vi "loadHTOutcounterOnly.vi"(10 "file path (dialog if empty)":path) -> ()   [LabVIEW 2012]
uses:
  <vilib>/addons/database/Connection.llb/DB Tools Open Connec (Path).vi
  <vilib>/Utility/file.llb/Read From Spreadsheet File (string).vi
  <vilib>/addons/database/Connection.llb/Conn Execute.vi
  <vilib>/addons/database/Recordset.llb/Rec Fetch Integer Data (R).vi
  <vilib>/addons/database/Recordset.llb/Rec Destroy - Connection.vi
  <vilib>/addons/database/NI_Database_API.lvlib
panel:
  out "ToRunSite":string
  out "error out 2":errorcluster
  in  "input cluster":T1
  out "output cluster":T1
  out "SQLDateTime":string
  out "time stamp":timestamp
  out "SQLDateTime 2":string
  out "concatenated string":string
  out "all rows":string[][](array[string])
  out "size(s)":i32[](array[numeric])
  out "output cluster 2":T2
  in  "input cluster 2":T2
  out "before substring 5":string
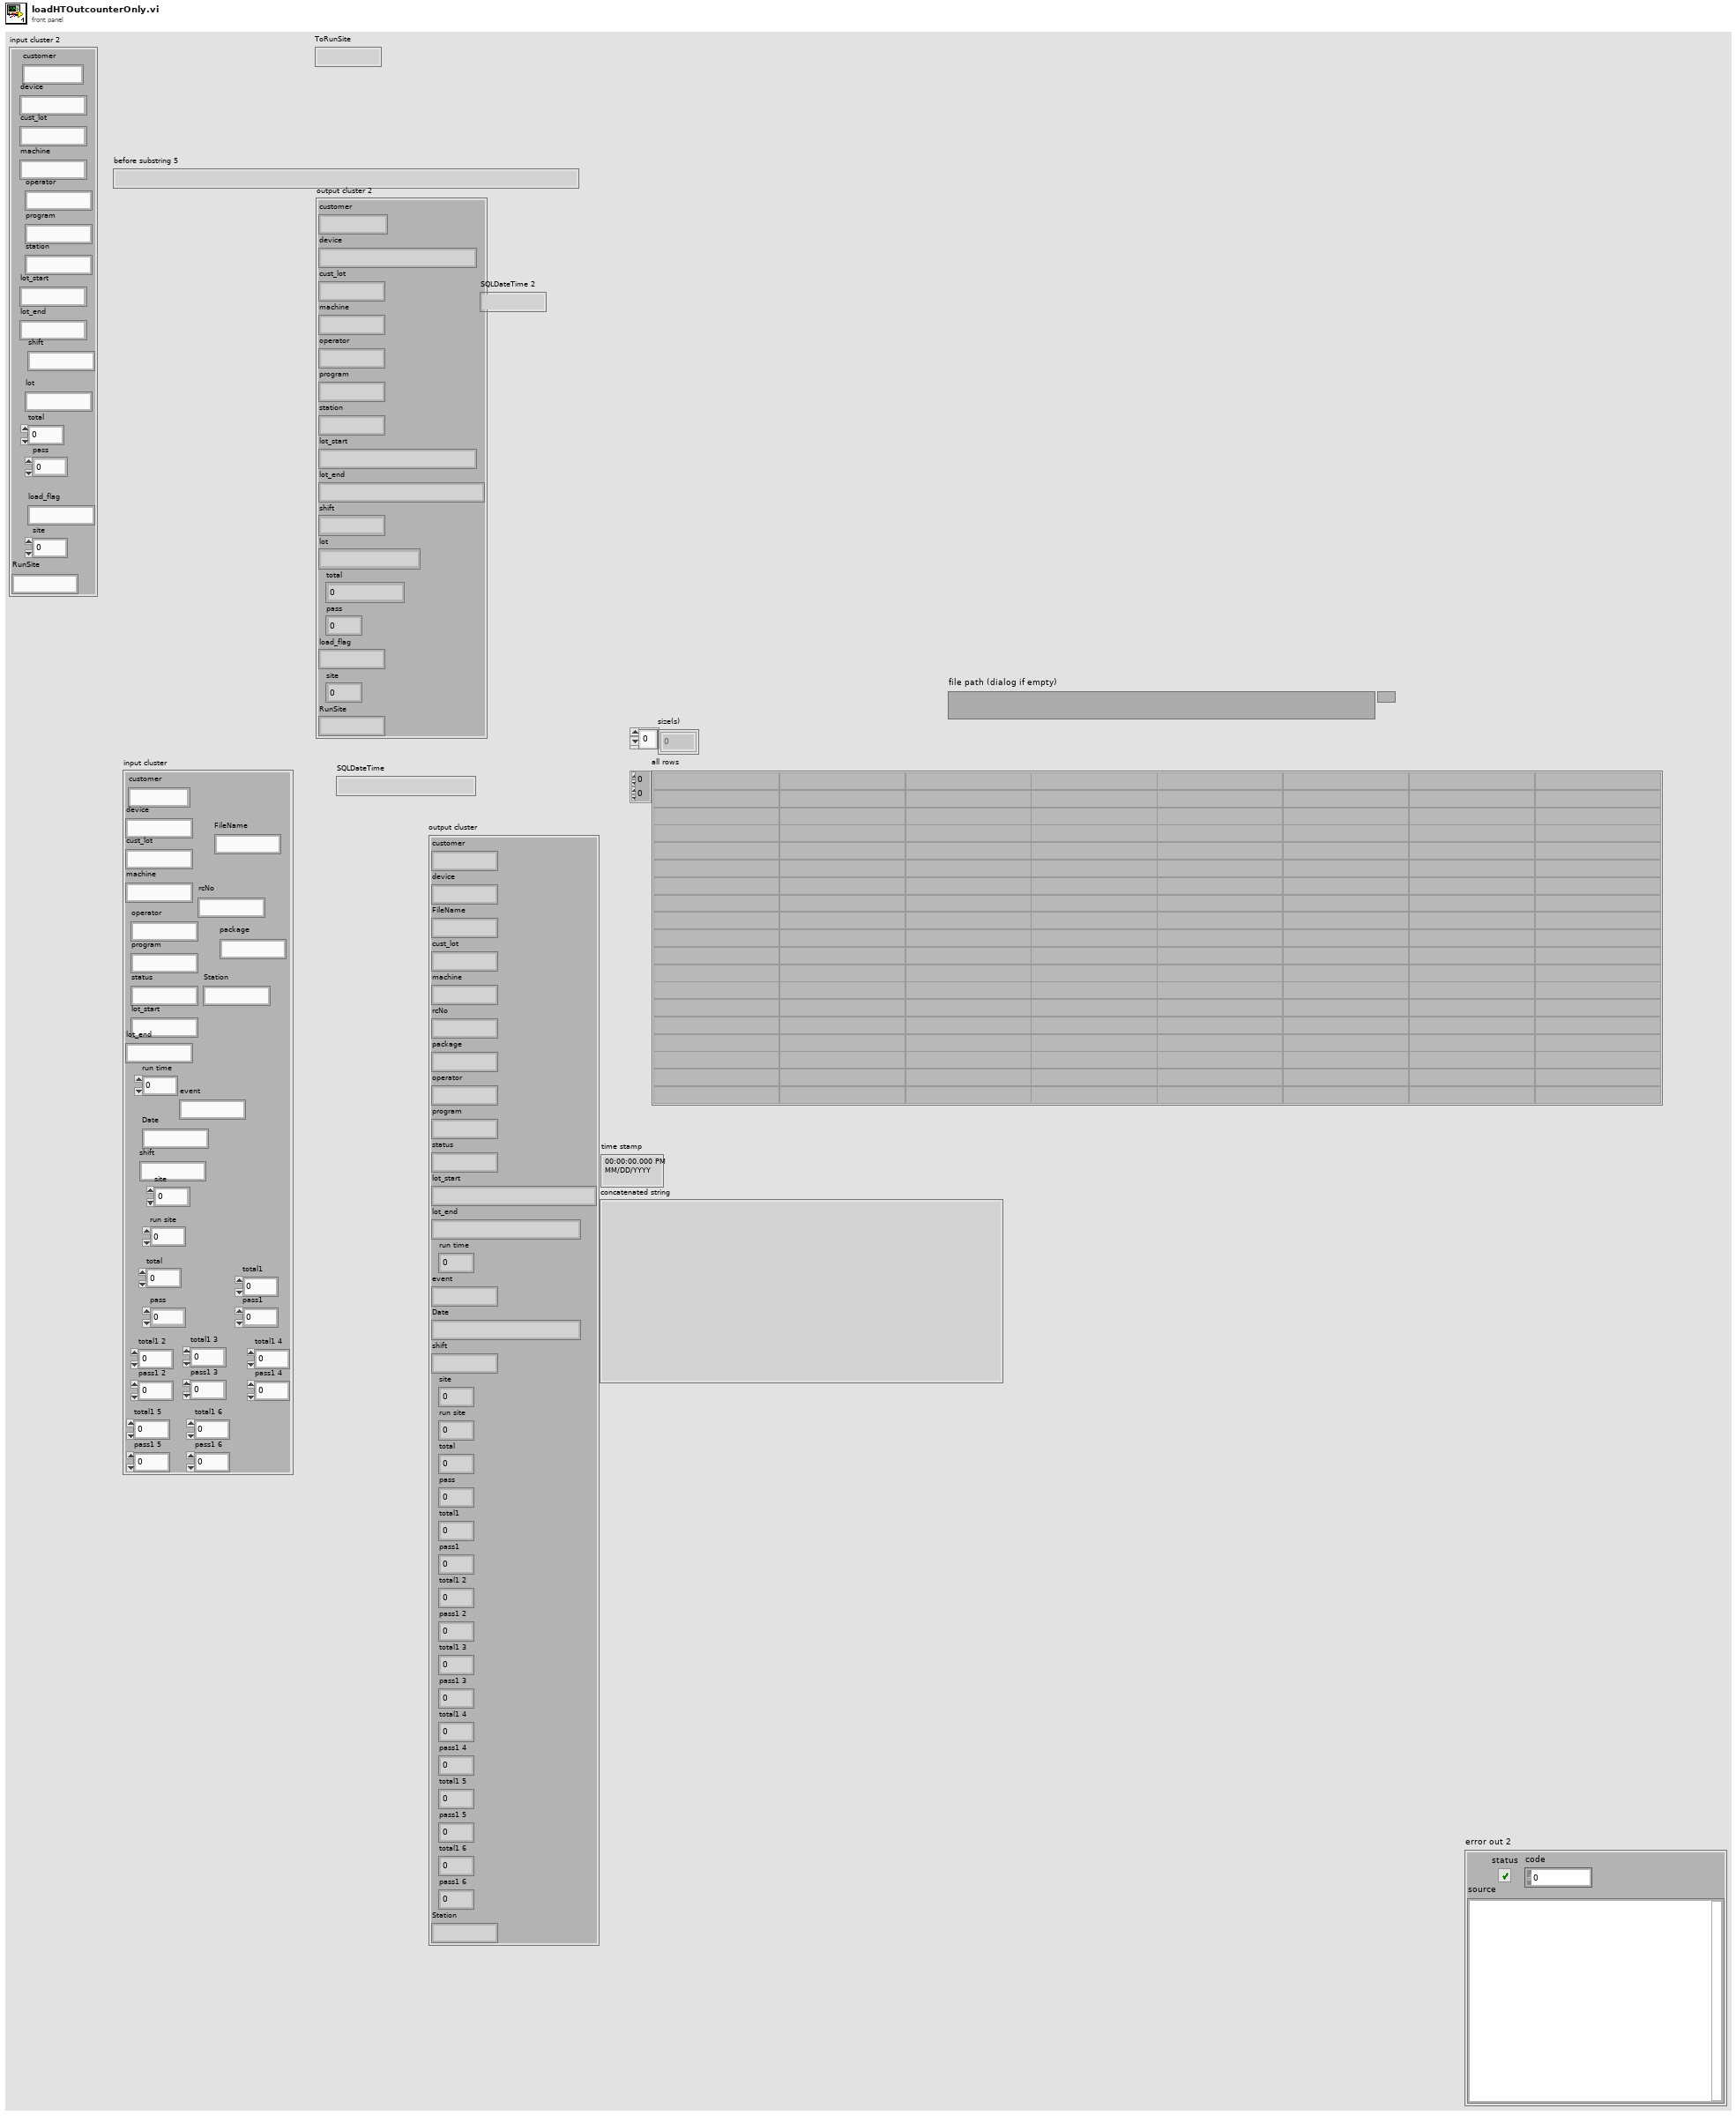
[diagram p1: front panel]
types:
  T1 = cluster{"customer":string, "device":string, "FileName":string, "cust_lot":string, "machine":string, "rcNo":string, "package":string, "operator":string, "program":string, "status":string, "lot_start":string, "lot_end":string, "run time":dbl, "event":string, "Date":string, "shift":string, "site":dbl, "run site ":dbl, "total":dbl, "pass":dbl, "total1":dbl, "pass1":dbl, "total1 2":dbl, "pass1 2":dbl, "total1 3":dbl, "pass1 3":dbl, "total1 4":dbl, "pass1 4":dbl, "total1 5":dbl, "pass1 5":dbl, "total1 6":dbl, "pass1 6":dbl, "Station":string}
  T2 = cluster{"customer":string, "device":string, "cust_lot":string, "machine":string, "operator":string, "program":string, "station":string, "lot_start":string, "lot_end":string, "shift":string, "lot":string, "total":dbl, "pass":dbl, "load_flag":string, "site":dbl, "RunSite":string}
  T3 = typedef "NI_Database_API.lvlib/Conn ObjectReference.ctl" = refnum<k1>
  T4 = typedef "NI_Database_API.lvlib/Rec ObjectReference.ctl" = refnum<k1>
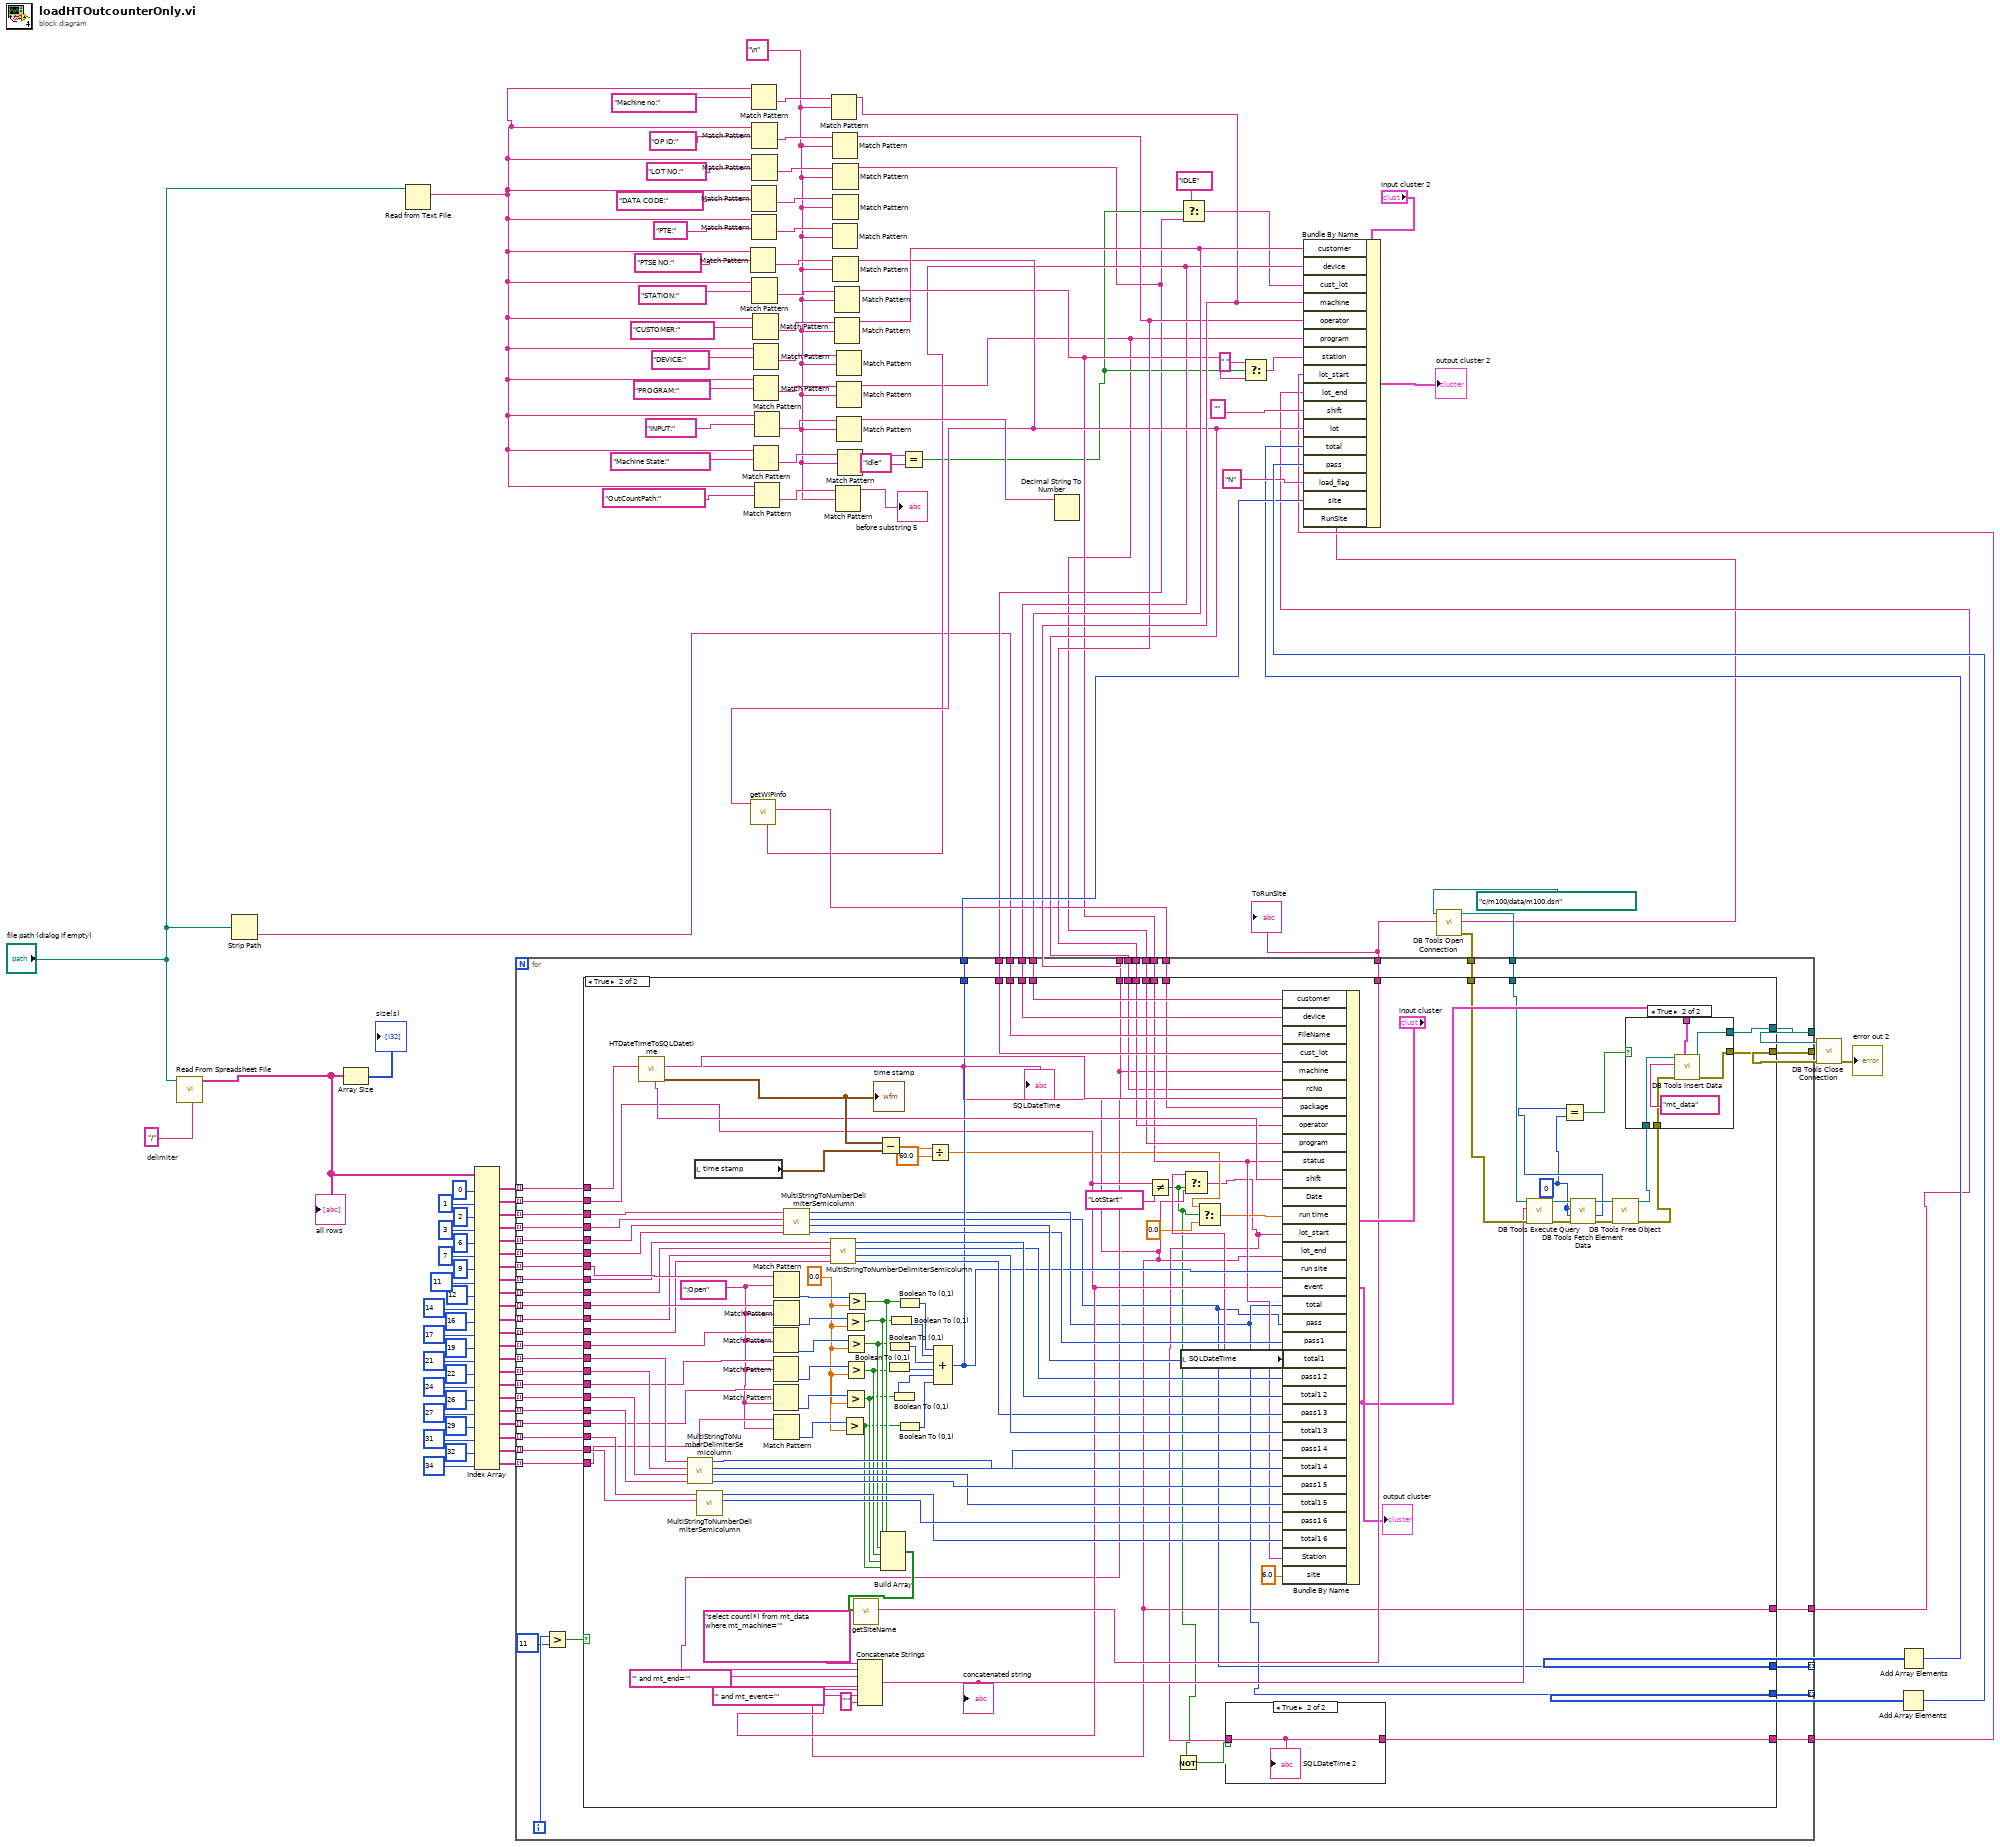
[diagram p0: block diagram]
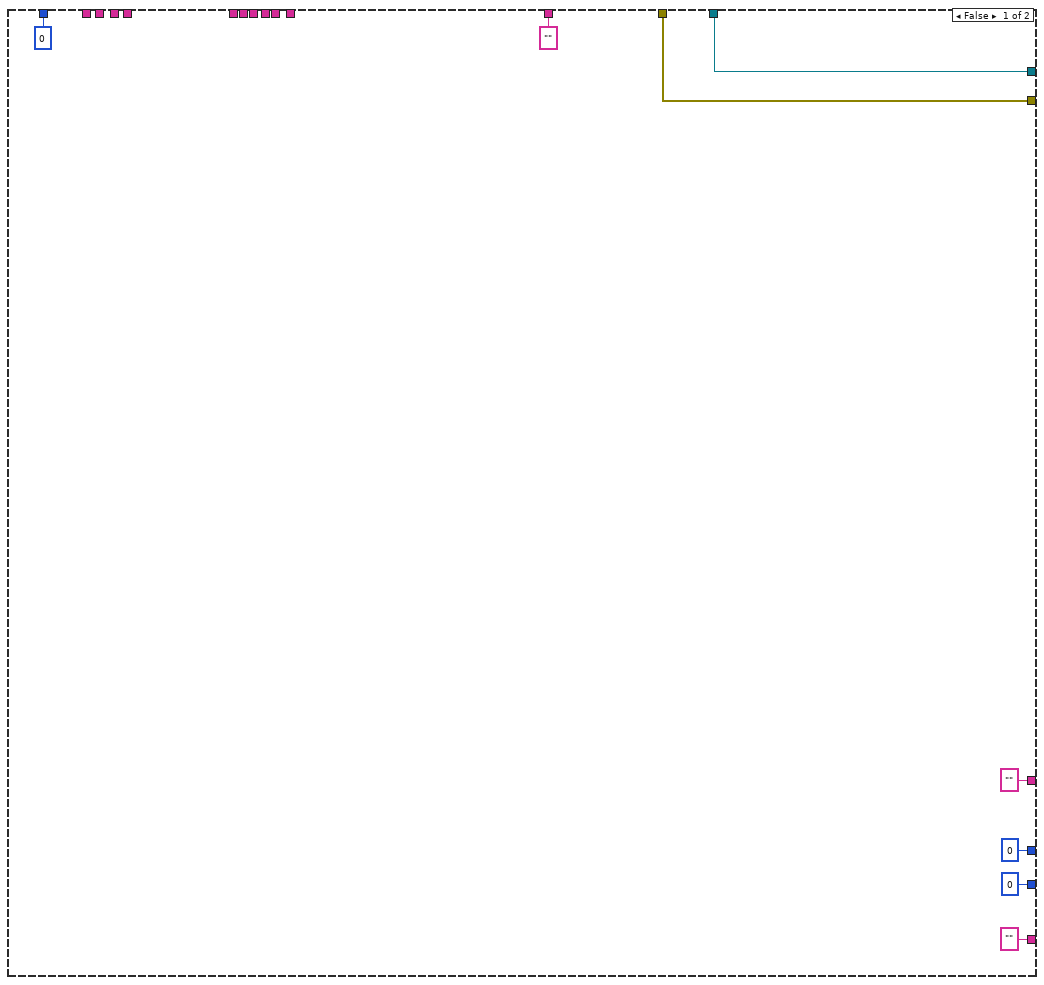
[diagram p2: hidden frame]
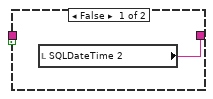
[diagram p4: hidden frame]
diagram:
  w80 = "/"  # delimiter
  w83 = "\n" ("regular expression")
  n1 = call-poly <vilib>:"Read From Spreadsheet File.vi"("delimiter (\\t)"=w80, "file path (dialog if empty)"="file path (dialog if empty)") -> ("all rows"=w78:string[][])  [unwired: 5 in, 4 out]
  "all rows" <- w78
  n2 = Strip Path(path="file path (dialog if empty)") -> (name=w2:string)  [unwired: 1 out]
  n3 = Array Size(array=w78) -> (size(s)=→"size(s)":i32[])
  n4 = Read from Text File(file (use dialog)="file path (dialog if empty)") -> (text=w81:string)  [unwired: 3 in, 3 out]
  n5 = Index Array(array=w78, index (col) #1=0 ("disabled index (col)"), index (col) #2=1 ("index (col)"), index (col) #3=2 ("index (col)"), index (col) #4=3 ("index (col)"), index (col) #5=6 ("index (col)"), index (col) #6=7 ("index (col)"), index (col) #7=9 ("index (col)"), index (col) #8=11 ("index (col)"), index (col) #9=12 ("index (col)"), index (col) #10=14 ("index (col)"), index (col) #11=16 ("index (col)"), index (col) #12=17 ("index (col)"), index (col) #13=19 ("index (col)"), index (col) #14=21 ("index (col)"), index (col) #15=22 ("index (col)"), index (col) #16=24 ("index (col)"), index (col) #17=26 ("index (col)"), index (col) #18=27 ("index (col)"), index (col) #19=29 ("index (col)"), index (col) #20=31 ("index (col)"), index (col) #21=32 ("index (col)"), index (col) #22=34 ("index (col)")) -> (element #1=w76:string[], element #2=w74:string[], element #3=w71:string[], element #4=w70:string[], element #5=w67:string[], element #6=w66:string[], element #7=w64:string[], element #8=w61:string[], element #9=w60:string[], element #10=w58:string[], element #11=w55:string[], element #12=w54:string[], element #13=w52:string[], element #14=w49:string[], element #15=w48:string[], element #16=w46:string[], element #17=w43:string[], element #18=w42:string[], element #19=w40:string[], element #20=w37:string[], element #21=w36:string[], element #22=w34:string[])  [unwired: 22 in]
  n6 = Match Pattern(string=w81, regular expression="PTSE NO:") -> (after substring=w104:string)  [unwired: 1 in, 3 out]
  n7 = Match Pattern(string=w81, regular expression="Machine no:") -> (after substring=w84:string)  [unwired: 1 in, 3 out]
  n8 = Match Pattern(string=w81, regular expression="DATA CODE:") -> (after substring=w108:string)  [unwired: 1 in, 3 out]
  n9 = Match Pattern(string=w81, regular expression="PTE:") -> (after substring=w106:string)  [unwired: 1 in, 3 out]
  n10 = Match Pattern(string=w81, regular expression="OP ID:") -> (after substring=w112:string)  [unwired: 1 in, 3 out]
  n11 = Match Pattern(string=w81, regular expression="LOT NO:") -> (after substring=w110:string)  [unwired: 1 in, 3 out]
  n12 = Match Pattern(string=w81, regular expression="STATION:") -> (after substring=w91:string)  [unwired: 1 in, 3 out]
  n13 = Match Pattern(string=w81, regular expression="CUSTOMER:") -> (after substring=w102:string)  [unwired: 1 in, 3 out]
  n14 = Match Pattern(string=w81, regular expression="DEVICE:") -> (after substring=w100:string)  [unwired: 1 in, 3 out]
  n15 = Match Pattern(string=w81, regular expression="PROGRAM:") -> (after substring=w98:string)  [unwired: 1 in, 3 out]
  n16 = Match Pattern(string=w81, regular expression="Machine State:") -> (after substring=w94:string)  [unwired: 1 in, 3 out]
  n17 = Match Pattern(string=w81, regular expression="INPUT:") -> (after substring=w96:string)  [unwired: 1 in, 3 out]
  n18 = Match Pattern(string=w81, regular expression="OutCountPath:") -> (after substring=w92:string)  [unwired: 1 in, 3 out]
  n19 = Match Pattern(string=w84, regular expression=w83) -> (before substring=w26:string)  [unwired: 1 in, 3 out]
  n20 = Match Pattern(string=w112, regular expression=w83) -> (before substring=w25:string)  [unwired: 1 in, 3 out]
  n21 = Match Pattern(string=w106, regular expression=w83) -> ()  [unwired: 1 in, 4 out]
  n22 = Match Pattern(string=w110, regular expression=w83) -> (before substring=w7:string)  [unwired: 1 in, 3 out]
  n23 = Match Pattern(string=w108, regular expression=w83) -> ()  [unwired: 1 in, 4 out]
  n24 = Match Pattern(string=w104, regular expression=w83) -> (before substring=w24:string)  [unwired: 1 in, 3 out]
  n25 = call "getWIPInfo.vi"("Lotno"=w24) -> ("Package"=w23:string, "Product"=w9:string)  [unwired: 4 in, 5 out]
  n26 = Match Pattern(string=w91, regular expression=w83) -> (before substring=w12:string)  [unwired: 1 in, 3 out]
  n27 = Match Pattern(string=w102, regular expression=w83) -> (before substring=w27:string)  [unwired: 1 in, 3 out]
  n28 = Match Pattern(string=w92, regular expression=w83) -> (before substring=→"before substring 5":string)  [unwired: 1 in, 3 out]
  n29 = Match Pattern(string=w100, regular expression=w83) -> ()  [unwired: 1 in, 4 out]
  n30 = Match Pattern(string=w98, regular expression=w83) -> (before substring=w4:string)  [unwired: 1 in, 3 out]
  n31 = Match Pattern(string=w96, regular expression=w83) -> (before substring=w86:string)  [unwired: 1 in, 3 out]
  n32 = Match Pattern(string=w94, regular expression=w83) -> (before substring=w14:string)  [unwired: 1 in, 3 out]
  n33 = Equal?(x=w14, y="Idle") -> (x = y?=w8:bool)
  n34 = Decimal String To Number(string=w86) -> ()  [unwired: 2 in, 2 out]
  n35 = Select(t="IDLE", s=w8, f=w7) -> (s? t:f=w6:string)
  n36 = Select(t=" ", s=w8, f=w12) -> (s? t:f=w11:string)
  n37 = call-poly <vilib>:"DB Tools Open Connection.vi"("connection information"=path "c:/m100/data/m100.dsn") -> ("error out"=w20:errorcluster, "connection reference"=w21:T3)  [unwired: 7 in]
  n38 = for {
    tunnel: w76 -> [w158] mode=indexing
    tunnel: w74 -> [w124] mode=indexing
    tunnel: w71 -> [w156] mode=indexing
    tunnel: w70 -> [w155] mode=indexing
    tunnel: w67 -> [w154] mode=indexing
    tunnel: w66 -> [w153] mode=indexing
    tunnel: w64 -> [w157] mode=indexing
    tunnel: w61 -> [w152] mode=indexing
    tunnel: w60 -> [w151] mode=indexing
    tunnel: w58 -> [w150] mode=indexing
    tunnel: w55 -> [w149] mode=indexing
    tunnel: w54 -> [w148] mode=indexing
    tunnel: w52 -> [w147] mode=indexing
    tunnel: w49 -> [w146] mode=indexing
    tunnel: w48 -> [w145] mode=indexing
    tunnel: w46 -> [w144] mode=indexing
    tunnel: w43 -> [w143] mode=indexing
    tunnel: w42 -> [w142] mode=indexing
    tunnel: w40 -> [w141] mode=indexing
    tunnel: w37 -> [w140] mode=indexing
    tunnel: w36 -> [w139] mode=indexing
    tunnel: w34 -> [w138] mode=indexing
    tunnel: [w120] -> w33 mode=indexing
    tunnel: [w129] -> w31
    tunnel: [w137] -> w3
    tunnel: [w119] -> w29 mode=indexing
    tunnel: w27 -> [w136]
    tunnel: w9 -> [w135]
    tunnel: w2 -> [w134]
    tunnel: w7 -> [w133]
    tunnel: w26 -> [w121]
    tunnel: w24 -> [w125]
    tunnel: w25 -> [w132]
    tunnel: w4 -> [w131]
    tunnel: w12 -> [w126]
    tunnel: w23 -> [w130]
    tunnel: w21 -> [w123]
    tunnel: w20 -> [w122]
    tunnel: [w128] -> w18
    tunnel: [w127] -> w17
    tunnel: [w118] -> w16
    tunnel: [w117] -> w15
    i -> [w116]
    n39 = Greater?(x=w116, y=11) -> (0:w114:bool)
    n40 = case shown="True" w114 {
      tunnel: w158 -> [_ w272]
      tunnel: w157 -> [_ w271]
      tunnel: w156 -> [_ w270]
      tunnel: w155 -> [_ w269]
      tunnel: w154 -> [_ w268]
      tunnel: w153 -> [_ w267]
      tunnel: w152 -> [_ w266]
      tunnel: w151 -> [_ w265]
      tunnel: w150 -> [_ w264]
      tunnel: w149 -> [_ w263]
      tunnel: w148 -> [_ w262]
      tunnel: w147 -> [_ w261]
      tunnel: w146 -> [_ w260]
      tunnel: w145 -> [_ w259]
      tunnel: w144 -> [_ w258]
      tunnel: w143 -> [_ w257]
      tunnel: w142 -> [_ w256]
      tunnel: w141 -> [_ w255]
      tunnel: w140 -> [_ w254]
      tunnel: w139 -> [_ w253]
      tunnel: w138 -> [_ w239]
      tunnel: ["" ("String") w211] -> w137
      tunnel: w136 -> [_ w210]
      tunnel: w135 -> [_ w209]
      tunnel: w134 -> [_ w208]
      tunnel: w133 -> [_ w207]
      tunnel: w132 -> [_ w206]
      tunnel: w131 -> [_ w205]
      tunnel: w130 -> [_ w204]
      tunnel: [i16 0 w203] -> w129
      tunnel: [w160 w202] -> w128
      tunnel: [w159 w201] -> w127
      tunnel: w126 -> [_ w198]
      tunnel: w125 -> [_ w193]
      tunnel: w124 -> [_ w192]
      tunnel: w123 -> [w160 w187]
      tunnel: w122 -> [w159 w186]
      tunnel: w121 -> [_ w179]
      tunnel: [0 ("number") w176] -> w120
      tunnel: [0 ("number 2") w175] -> w119
      tunnel: ["" ("SQLDateTime") w171] -> w118
      tunnel: ["" ("SQLDateTime") w170] -> w117
      frame False {
      }
      frame True {
        w183 = 0
        w231 = 0.0 ("y")
        w238 = ":Open" ("regular expression")
        n41 = call "HTDateTimeToSQLDatetime.vi"("HTDateTime"=w272) -> ("time stamp"=w223:timestamp, "date string"=w220:string, "SQLDateTime"=w170:string, "Shift"=w219:string)  [unwired: 7 in]
        "SQLDateTime" <- w170
        "time stamp" <- w223
        n42 = call "MultiStringToNumberDelimiterSemicolumn.vi"("input string 4"=w256, "input string 3"=w257, "input string 2"=w259, "input string"=w260) -> ("number 4"=w249:i32, "number 3"=w248:i32, "number 2"=w247:i32, "number"=w246:i32)  [unwired: 4 in]
        n43 = local read "time stamp"() -> (w224:timestamp)
        n44 = call "MultiStringToNumberDelimiterSemicolumn.vi"("input string 2"=w253, "input string"=w254) -> ("number 2"=w251:i32, "number"=w250:i32)  [unwired: 6 in, 2 out]
        n45 = Match Pattern(string=w261, regular expression=w238) -> (offset past match=w235:i32)  [unwired: 1 in, 3 out]
        n46 = Match Pattern(string=w258, regular expression=w238) -> (offset past match=w234:i32)  [unwired: 1 in, 3 out]
        n47 = Match Pattern(string=w255, regular expression=w238) -> (offset past match=w233:i32)  [unwired: 1 in, 3 out]
        n48 = Match Pattern(string=w271, regular expression=w238) -> (offset past match=w237:i32)  [unwired: 1 in, 3 out]
        n49 = Match Pattern(string=w264, regular expression=w238) -> (offset past match=w236:i32)  [unwired: 1 in, 3 out]
        n50 = Match Pattern(string=w239, regular expression=w238) -> (offset past match=w232:i32)  [unwired: 1 in, 3 out]
        n51 = call "MultiStringToNumberDelimiterSemicolumn.vi"("input string 4"=w267, "input string 3"=w268, "input string 2"=w269, "input string"=w270) -> ("number 4"=w240:i32, "number 3"=w241:i32, "number 2"=w175:i32, "number"=w176:i32)  [unwired: 4 in]
        n52 = call "MultiStringToNumberDelimiterSemicolumn.vi"("input string 4"=w262, "input string 3"=w263, "input string 2"=w265, "input string"=w266) -> ("number 4"=w244:i32, "number 3"=w245:i32, "number 2"=w242:i32, "number"=w243:i32)  [unwired: 4 in]
        n53 = Greater?(x=w232, y=w231) -> (0:w213:bool)
        n54 = Greater?(x=w236, y=w231) -> (0:w217:bool)
        n55 = Greater?(x=w233, y=w231) -> (0:w214:bool)
        n56 = Greater?(x=w235, y=w231) -> (0:w216:bool)
        n57 = Greater?(x=w234, y=w231) -> (0:w215:bool)
        n58 = Greater?(x=w237, y=w231) -> (0:w218:bool)
        n59 = Concatenate Strings("select count(*) from mt_data where mt_machine='" ("string"), w179, "' and mt_end='" ("string"), w170, "' and mt_event='" ("string"), w192, "'" ("string")) -> (w185:string)
        "concatenated string" <- w185
        n60 = Subtract(x=w223, y=w224) -> (x-y=w222:dbl)
        n61 = Build Array(w218, w217, w216, w215, w214, w213) -> (w212:bool[])
        n62 = call "getSiteName.vi"("Array"=w212) -> ("String"=w211:string)  [unwired: 10 in]
        n63 = Boolean To (0,1)(Boolean=w215) -> (0, 1=w227:i16)
        n64 = Boolean To (0,1)(Boolean=w216) -> (0, 1=w228:i16)
        n65 = Boolean To (0,1)(Boolean=w217) -> (0, 1=w229:i16)
        n66 = Boolean To (0,1)(Boolean=w214) -> (0, 1=w226:i16)
        n67 = Boolean To (0,1)(Boolean=w218) -> (0, 1=w230:i16)
        n68 = Boolean To (0,1)(Boolean=w213) -> (0, 1=w225:i16)
        n69 = Divide(x=w222, y=60.0) -> (x/y=w174:dbl)
        n70 = Compound Arithmetic op=ADD(w230, w229, w228, w227, w226, w225) -> (w203:i16)
        n71 = Not Equal?(x=w192, y="LotStart") -> (x != y?=w168:bool)
        n72 = Not(x=w168) -> (.not. x?=w167:bool)
        n73 = local read "SQLDateTime"() -> (w177:string)
        n74 = Select(t=w177, s=w168, f=w170) -> (s? t:f=w172:string)
        n75 = Select(t=w174, s=w168, f=0.0 ("t")) -> (s? t:f=w178:dbl)
        n76 = case shown="True" w167 {
          tunnel: w172 -> [_ w282]
          tunnel: [w281 w282] -> w171
          frame False {
            n77 = local read "SQLDateTime 2"() -> (w281:string)
          }
          frame True {
            "SQLDateTime 2" <- w282
          }
        }
        n78 = Bundle By Name(cluster="input cluster", "customer"=w210, "device"=w209, "FileName"=w208, "cust_lot"=w207, "machine"=w179, "rcNo"=w193, "package"=w204, "operator"=w206, "program"=w205, "status"=w198, "shift"=w219, "Date"=w220, "run time"=w178, "lot_start"=w172, "lot_end"=w170, "run site"=w203, "event"=w192, "total"=w176, "pass"=w175, "pass1"=w240, "total1"=w241, "pass1 2"=w242, "total1 2"=w243, "pass1 3"=w244, "total1 3"=w245, "pass1 4"=w247, "total1 4"=w246, "pass1 5"=w249, "total1 5"=w248, "pass1 6"=w251, "total1 6"=w250, "Station"=w198, "site"=6.0) -> (w200:T1)
        "output cluster" <- w200
        n79 = call-poly <vilib>:"DB Tools Execute Query.vi"("error in (no error)"=w186, "SQL query"=w185, "connection reference"=w187) -> ("error out"=w191:errorcluster, "recordset reference"=w190:T4)  [unwired: 5 in]
        n80 = call-poly <vilib>:"DB Tools Fetch Element Data.vi"("error in (no error)"=w191, "type"=w183, "column index"=w183, "recordset reference"=w190) -> ("error out"=w189:errorcluster, "data"=w184:i32, "recordset reference out"=w188:T4)  [unwired: 3 in]
        n81 = Equal?(x=w184, y=w183) -> (x = y?=w182:bool)
        n82 = call-poly <vilib>:"DB Tools Free Object.vi"("error in (no error)"=w189, "recordset reference"=w188) -> ("error out"=w180:errorcluster, "connection reference"=w181:T3)  [unwired: 8 in]
        n83 = case shown="True" w182 {
          tunnel: [w274 w280] -> w202
          tunnel: [w273 w279] -> w201
          tunnel: w200 -> [_ w277]
          tunnel: w181 -> [w274 w276]
          tunnel: w180 -> [w273 w275]
          frame False {
          }
          frame True {
            n84 = call <vilib>:"DB Tools Insert Data.vi"("data"=w277, "error in (no error)"=w275, "table"="mt_data", "connection reference"=w276) -> ("error out"=w279:errorcluster, "connection reference out"=w280:T3)  [unwired: 6 in]
          }
        }
      }
    }
  }
  "ToRunSite" <- w3
  n85 = call <vilib>:"DB Tools Close Connection.vi"("error in (no error)"=w17, "connection reference"=w18) -> ("error out"=→"error out 2":errorcluster)  [unwired: 5 in]
  n86 = Add Array Elements(numeric array=w33) -> (sum=w32:i32)
  n87 = Add Array Elements(numeric array=w29) -> (sum=w28:i32)
  n88 = Bundle By Name(cluster="input cluster 2", "customer"=w27, "device"=w9, "cust_lot"=w6, "machine"=w26, "operator"=w25, "program"=w4, "station"=w11, "lot_start"=w16, "lot_end"=w15, "shift"="" ("lot_end"), "lot"=w24, "total"=w28, "pass"=w32, "load_flag"="N", "site"=w31, "RunSite"=w3) -> (→"output cluster 2":T2)
